vi "Fill_Fruit_Box.vi"() -> (5 "Plug in titles":string[](array[string]), 7 "Plug in values":string[](array[string]))   [LabVIEW 2010]
uses:
  Controls/Post_Process.ctl
  Globals/Meas_global.vi
  Globals/Dynamic_call_global.ph.vi
panel:
  out "Case Currently On":string
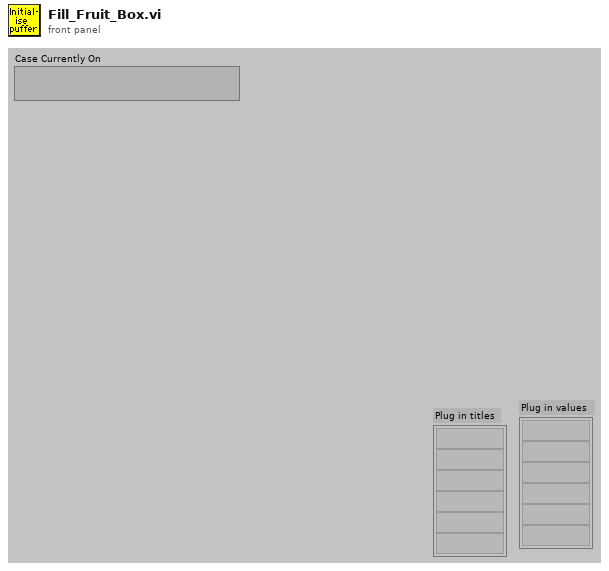
[diagram p1: front panel]
types:
  T1 = typedef "Post_Process.ctl" = enum16{"Take New Data", "Post Process Raw Data File"}
  T2 = typedef "Rendezvous RefNum" = refnum<k1>
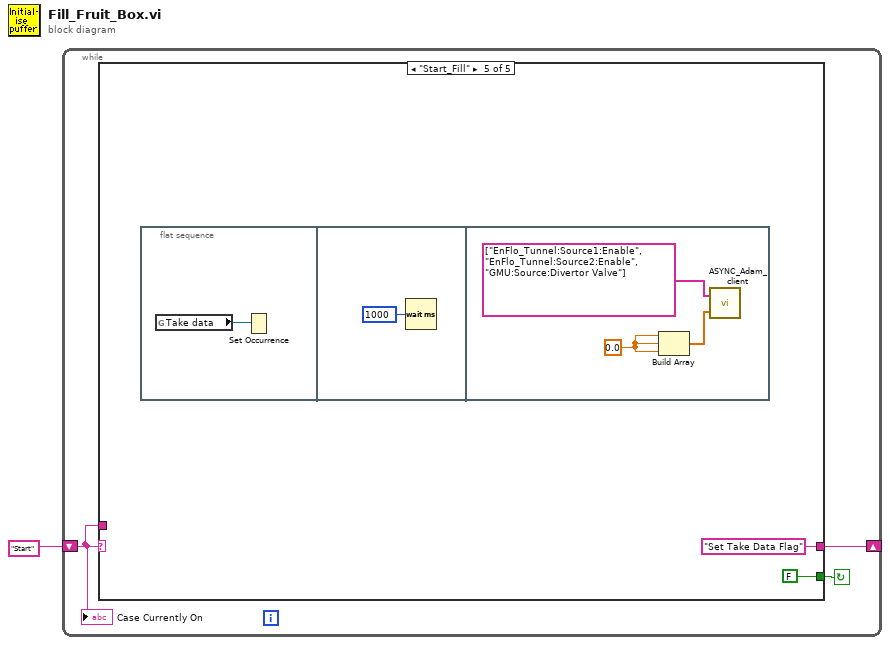
[diagram p0: block diagram]
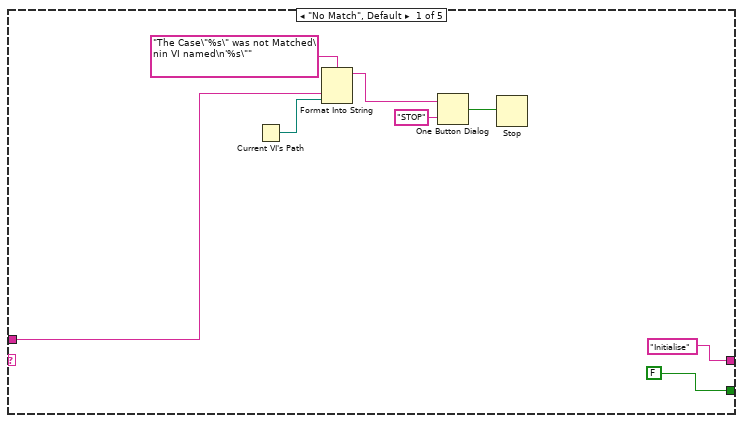
[diagram p2: hidden frame]
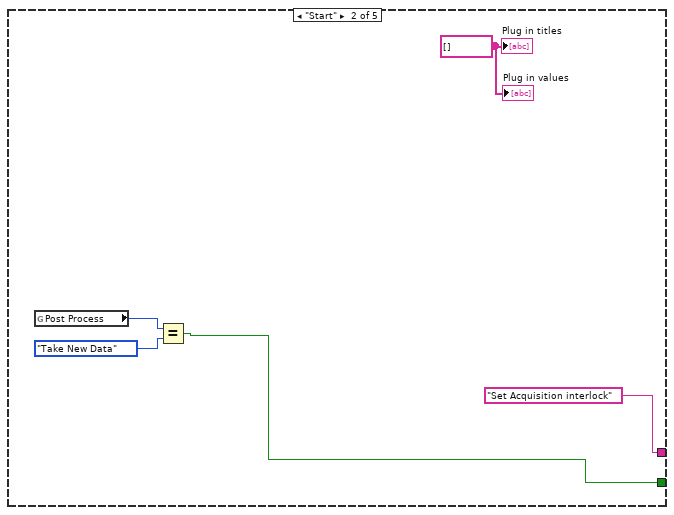
[diagram p3: hidden frame]
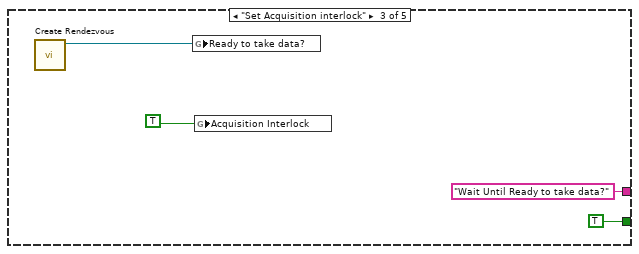
[diagram p4: hidden frame]
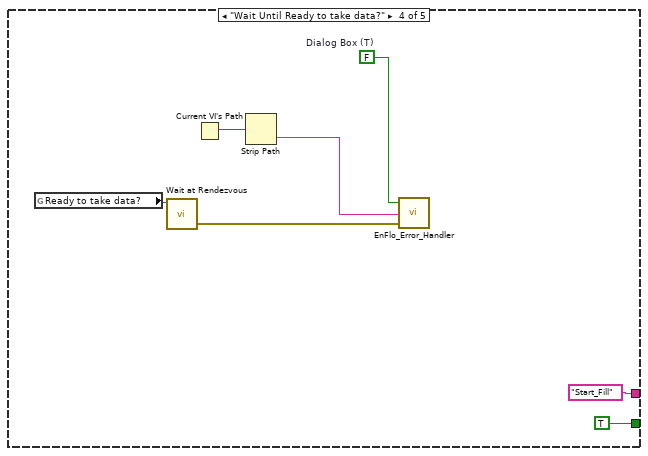
[diagram p5: hidden frame]
diagram:
  n1 = while {
    shift-left: "Start" -> [w2]
    shift-right: [w3] -> _
    stop <- w4 continue-if-true
    n2 = case shown="\"Start_Fill\"" w2 {
      tunnel: [FALSE w13 TRUE ("Command Found") TRUE ("Command Found") FALSE ("Command Found")] -> w4
      tunnel: ["Initialise" "Set Acquisition interlock" "Wait Until Ready to take data?" "Start_Fill" "Set Take Data Flag"] -> w3
      tunnel: w2 -> [w7 _ _ _ _]
      frame "No Match", Default {
        n3 = Current VI's Path() -> (path=w6:path)
        n4 = Format Into String(format string="The Case\"%s\" was not Matched\nin VI named\n'%s\"" ("Format String"), w7, w6) -> (resulting string=w10:string)  [unwired: 2 in, 1 out]
        n5 = One Button Dialog(message=w10, button name ("OK")="STOP") -> (true=w8:bool)
        n6 = Stop(stop? (T)=w8) -> ()
      }
      frame "Start" {
        w14 = string[] [] ("Plug in titles")
        n7 = global read "Meas_global.vi" "Post Process"() -> (w15:T1)
        n8 = Equal?(x=w15, y=Post_Process."Take New Data" ("Post Process")) -> (x = y?=w13:bool)
        "Plug in values" <- w14
        "Plug in titles" <- w14
      }
      frame "Set Acquisition interlock" {
        n9 = call <vilib>:"Create Rendezvous.vi"() -> ("rendezvous"=w18:T2)  [unwired: 5 in, 2 out]
        n10 = global write "Dynamic_call_global.ph.vi" "Ready to take data?"(w18) -> ()
        n11 = global write "Dynamic_call_global.ph.vi" "Acquisition Interlock"(TRUE ("Remote control")) -> ()
      }
      frame "Wait Until Ready to take data?" {
        w24 = FALSE  # Dialog Box (T)
        n12 = global read "Dynamic_call_global.ph.vi" "Ready to take data?"() -> (w27:T2)
        n13 = call <vilib>:"Wait at Rendezvous.vi"("rendezvous"=w27) -> ("error out"=w25:errorcluster)  [unwired: 4 in, 2 out]
        n14 = Current VI's Path() -> (path=w23:path)
        n15 = Strip Path(path=w23) -> (name=w22:string)  [unwired: 1 out]
        n16 = call "EnFlo_Error_Handler.vi"("error in (no error)"=w25, "Error Type"=w22, "Dialog Box (T)"=w24) -> ()  [unwired: 3 out]
      }
      frame "Start_Fill" {
        n17 = flat-sequence {
          frame #0 {
            n18 = global read "Dynamic_call_global.ph.vi" "Take data"() -> (w31:refnum<k4>)
            n19 = Set Occurrence(w31) -> ()
          }
          frame #1 {
            n20 = Wait (ms)(milliseconds to wait=u32 1000) -> ()  [unwired: 1 out]
          }
          frame #2 {
            w33 = 0.0 ("New Value")
            n21 = Build Array(w33, w33, w33) -> (w35:dbl[])
            n22 = call "ASYNC_Adam_client.vi"("Values"=w35, "Channel Names"=string[] ["EnFlo_Tunnel:Source1:Enable", "EnFlo_Tunnel:Source2:Enable", "GMU:Source:Divertor Valve"] ("appended array")) -> ()  [unwired: 2 out]
          }
        }
      }
    }
    "Case Currently On" <- w2
  }
